vi "SG_output.vi"(7 "Func.":enum16{"Disable", "Enable"}(ring), 8 "error in":errorcluster, 11 "VISA in":refnum<visa-resource-name>) -> (0 "error out":errorcluster, 3 "VISA out":refnum<visa-resource-name>)   [LabVIEW 2023, in "Keysight.lvlib"]
uses:
  Keysight.lvlib
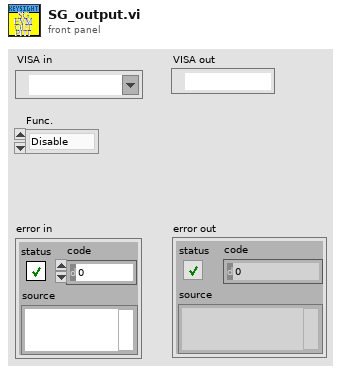
[diagram p1: front panel]
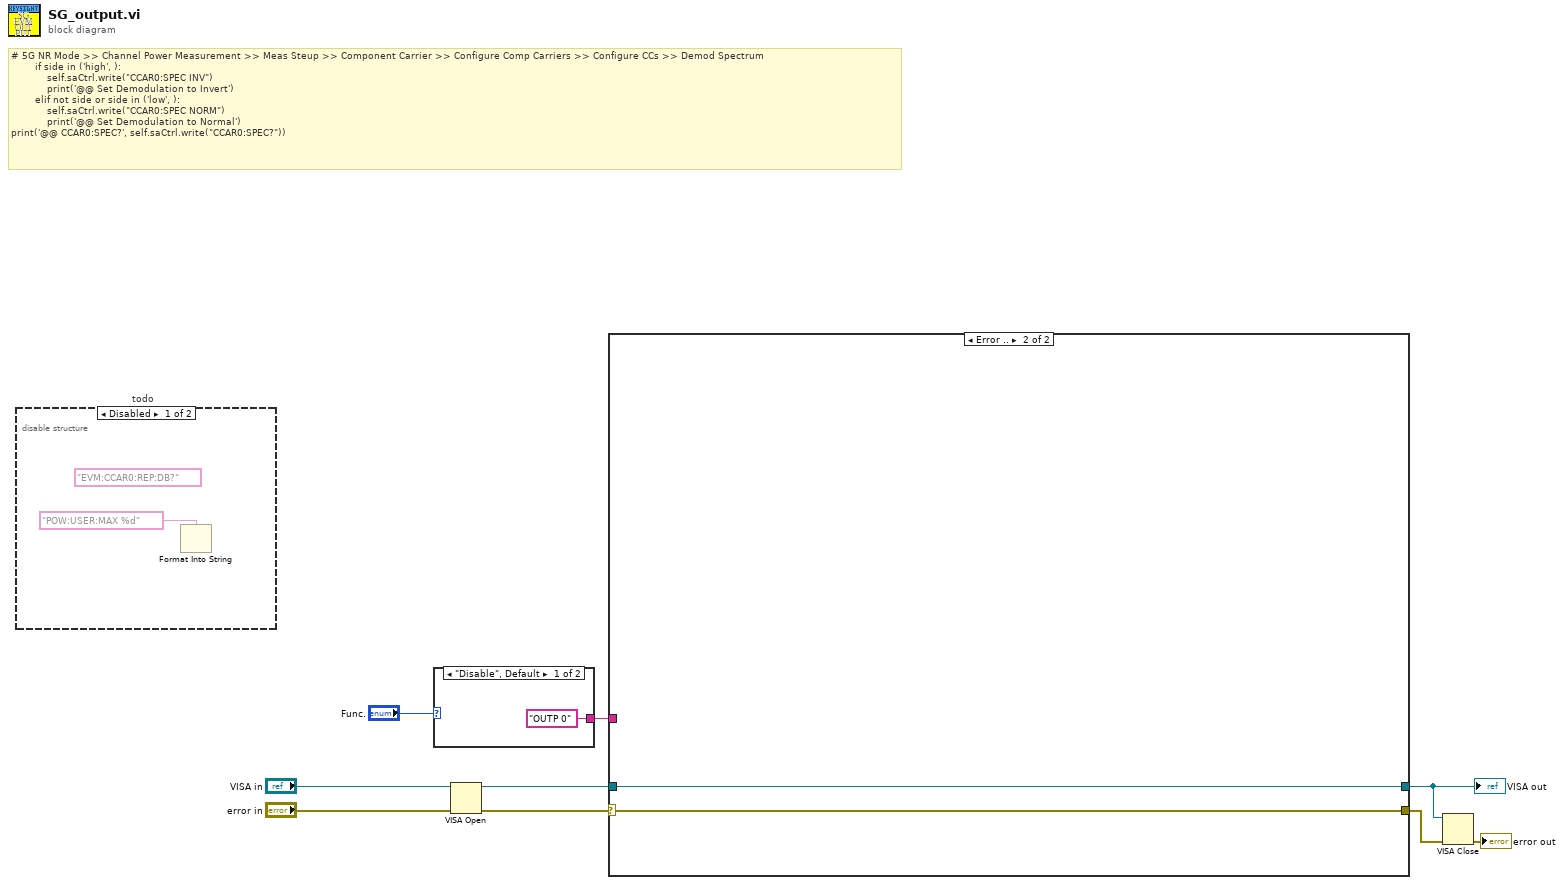
[diagram p0: block diagram]
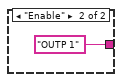
[diagram p2: hidden frame]
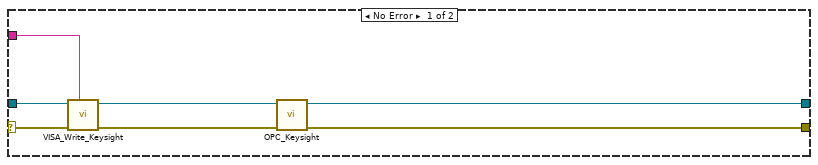
[diagram p4: hidden frame]
diagram:
  # "# 5G NR Mode >> Channel Power Measurement >> Meas Steup >> Component Carrier >> Configure Comp Carriers >> Configure CCs >> Demod Spectrum\n        if side in ('high', ):\n            self.saCtrl.write(\"CCAR0:SPEC INV\")\n            print('@@ Set Demodulation to Invert')\n        elif not side or side in ('low', ):\n            self.saCtrl.write(\"CCAR0:SPEC NORM\")\n            print('@@ Set Demodulation to Normal')\nprint('@@ CCAR0:SPEC?', self.saCtrl.write(\"CCAR0:SPEC?\"))"
  n1 = disable-structure "todo" shown="Disabled" {
    frame Disabled {
      (unwired) "EVM:CCAR0:REP:DB?" ("write buffer")
      n2 = Format Into String(format string="POW:USER:MAX %d") -> ()  [unwired: 3 in, 2 out]
    }
    frame Enabled {
    }
  }
  n3 = case shown="\"Disable\", Default" "Func." {
    tunnel: ["OUTP 0" ("write buffer") "OUTP 1" ("write buffer")] -> w9
    frame "Disable", Default {
    }
    frame "Enable" {
    }
  }
  n4 = VISA Open(error in (no error)="error in", VISA resource name="VISA in") -> (VISA resource name=w7:refnum<visa-resource-name>, error out=w6:errorcluster)  [unwired: 3 in]
  n5 = case shown="Error .." w6 {
    selector: w6 -> [w19 w20]
    tunnel: w7 -> [w18 w21]
    tunnel: w9 -> [w17 _]
    tunnel: [w16 w20] -> w5
    tunnel: [w15 w21] -> w3
    frame No Error {
      n6 = call "VISA_Write_Keysight.vi"("VISA CMD"=w17, "error in"=w19, "VISA in"=w18) -> ("error out"=w13:errorcluster, "VISA out"=w14:refnum<visa-resource-name>)  [unwired: 7 in]
      n7 = call "OPC_Keysight.vi"("error in (no error)"=w13, "VISA resource name"=w14) -> ("error out"=w16:errorcluster, "VISA resource name out"=w15:refnum<visa-resource-name>)  [unwired: 8 in]
    }
    frame Error {
    }
  }
  "VISA out" <- w3
  n8 = VISA Close(VISA resource name=w3, error in (no error)=w5) -> (error out=→"error out":errorcluster)
